vi "MenuOptions.vi"(8 "error in":errorcluster, 10 "VI ref":refnum<vi>, 11 "menu ref in":refnum<k9>) -> (0 "error out":errorcluster, 3 "menu ref out":refnum<k9>)   [LabVIEW 2025, in "Config Tool.lvlib"]
doc: "This VI configures the application menu options. If you need aditional menu items add them in this VI.Copyright 2017 National Instruments Corporation\n\nLicensed under the Apache License, Version 2.0 (the \"License\"); you may not use this file except in compliance with the License. You may obtain a copy of the License at http://www.apache.org/licenses/LICENSE-2.0\nUnless required by applicable law or agreed to in writing, software distributed under the License is distributed on an \"AS IS\" BASIS, WITHOUT WARRANTIES OR CONDITIONS OF ANY KIND, either express or implied. See the License for the specific language governing permissions and limitations under the License."
uses:
  Config Tool.lvlib
  <vilib>/Utility/miscctls.llb/LVMenuShortCut.ctl
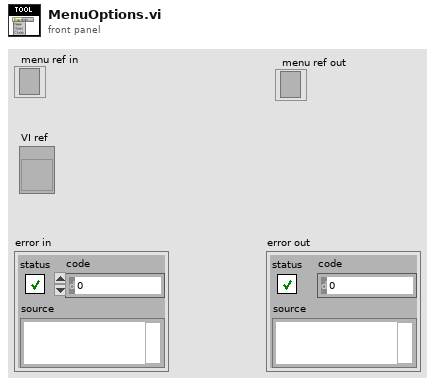
[diagram p1: front panel]
types:
  T1 = typedef "LVMenuShortCut.ctl" = cluster{"Include Shift Key?":bool, "Include Ctrl Key?":bool, "Shortcut Key":string}
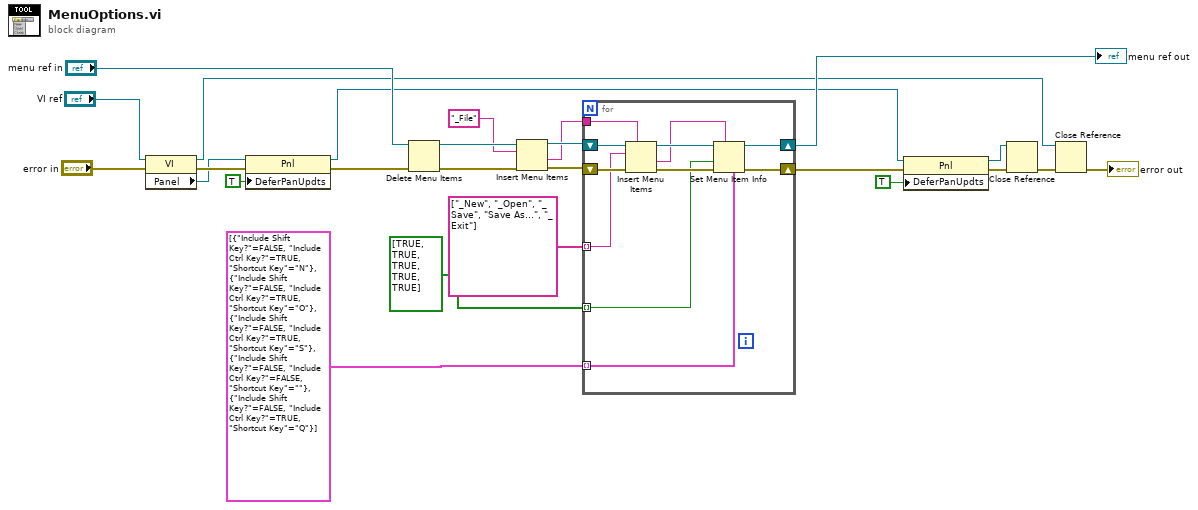
[diagram p0: block diagram]
diagram:
  n1 = property class="VI"(reference="VI ref", error in="error in") -> (reference out=w1:refnum<vi>, error out=w14:errorcluster, "Panel"=w13:refnum<vi>)
  n2 = property class="Pnl"(reference=w13, error in=w14, "DeferPanUpdts"=TRUE ("Defer Panel Updates")) -> (reference out=w4:refnum<vi>, error out=w9:errorcluster)
  n3 = Delete Menu Items(6:w9, 9:"menu ref in") -> (0:w21:errorcluster, 3:w24:refnum<k9>)  [unwired: 2 in]
  n4 = Insert Menu Items(6:w21, 8:"_File", 9:w24) -> (0:w20:errorcluster, 1:w17:string, 3:w22:refnum<k9>)  [unwired: 3 in]
  n5 = for {
    shift-right: [w36] -> w16
    shift-left: w22 -> [w31]
    tunnel: T1[] [{"Include Shift Key?"=FALSE, "Include Ctrl Key?"=TRUE, "Shortcut Key"="N"}, {"Include Shift Key?"=FALSE, "Include Ctrl Key?"=TRUE, "Shortcut Key"="O"}, {"Include Shift Key?"=FALSE, "Include Ctrl Key?"=TRUE, "Shortcut Key"="S"}, {"Include Shift Key?"=FALSE, "Include Ctrl Key?"=FALSE, "Shortcut Key"=""}, {"Include Shift Key?"=FALSE, "Include Ctrl Key?"=TRUE, "Shortcut Key"="Q"}] -> [w34] mode=indexing
    shift-right: [w35] -> w3
    shift-left: w20 -> [w33]
    tunnel: string[] ["_New", "_Open", "_Save", "Save As...", "_Exit"] ("item names") -> [w29] mode=indexing
    tunnel: w17 -> [w28]
    tunnel: bool[] [TRUE, TRUE, TRUE, TRUE, TRUE] -> [w26] mode=indexing
    n6 = Insert Menu Items(5:w28, 6:w33, 8:w29, 9:w31) -> (0:w32:errorcluster, 1:w27:string, 3:w30:refnum<k9>)  [unwired: 2 in]
    n7 = Set Menu Item Info(4:w34, 7:w27, 8:w32, 9:w26, 11:w30) -> (0:w35:errorcluster, 3:w36:refnum<k9>)  [unwired: 2 in]
  }
  "menu ref out" <- w16
  n8 = property class="Pnl"(reference=w4, error in=w3, "DeferPanUpdts"=TRUE ("Defer Panel Updates")) -> (reference out=w2:refnum<vi>, error out=w7:errorcluster)
  n9 = Close Reference(reference=w2, error in (no error)=w7) -> (error out=w8:errorcluster)
  n10 = Close Reference(reference=w1, error in (no error)=w8) -> (error out=→"error out":errorcluster)
